vi "MarkMeasResult.vi"(4 "error in (no error)":errorcluster, 5 "Data useful?":i32(ring) items=["No", "Yes"], 6 "measResId":i32, 7 "Database":T1={"DB name"="zaop", "UID"="", "password"=""}) -> (0 "error out":errorcluster)   [LabVIEW 2016]
doc: "Marks a result set as usable or unusable, updating the field \"isDataUsable\" in the database table meas_res_summary for the given measResId. The input \"Data useful?\" is 1 for yes, 0 for no."
uses:
  type def/Database.ctl
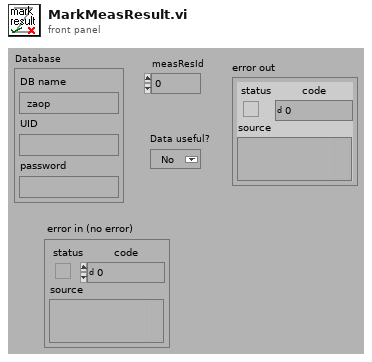
[diagram p1: front panel]
types:
  T1 = typedef "Database.ctl" = cluster{"DB name":string, "UID":string, "password":string}
  T2 = typedef "Connection - Recordset reference.ctl" = cluster{"Connection":refnum<k7>, "Recordset":refnum<k7>}
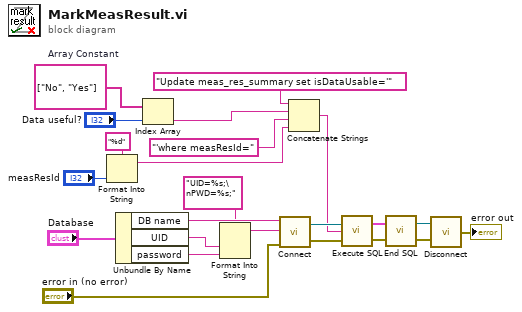
[diagram p0: block diagram]
diagram:
  w13 = string[] ["No", "Yes"]  # Array Constant
  n1 = Format Into String(format string="%d" ("Format String"), "measResId") -> (resulting string=w6:string)  [unwired: 2 in, 1 out]
  n2 = Unbundle By Name("Database") -> ("DB name"=w19:string, "UID"=w22:string, "password"=w21:string)
  n3 = Index Array(array=w13, index="Data useful?") -> (element=w10:string)
  n4 = Format Into String(format string="UID=%s;\nPWD=%s;" ("Format String"), w22, w21) -> (resulting string=w20:string)  [unwired: 2 in, 1 out]
  n5 = call <vilib>:"Connect.vi"("error in (no error)"="error in (no error)", "connection parameters"=w20, "data source name"=w19) -> ("error out"=w15:errorcluster, "Connection"=w16:refnum<k7>)  [unwired: 1 in]
  n6 = Concatenate Strings("Update meas_res_summary set isDataUsable='" ("Substring"), w10, "'where measResId=" ("Substring"), w6) -> (w3:string)
  n7 = call <vilib>:"Execute SQL.vi"("error in (no error)"=w15, "SQL Statement"=w3, "Connection"=w16) -> ("error out"=w17:errorcluster, "reference"=w18:T2)
  n8 = call <vilib>:"End SQL.vi"("error in (no error)"=w17, "reference"=w18) -> ("error out"=w4:errorcluster, "Connection"=w5:refnum<k7>)
  n9 = call <vilib>:"Disconnect.vi"("error in (no error)"=w4, "connection"=w5) -> ("error out"=→"error out":errorcluster)  [unwired: 1 in]
